vi "Display.vi"() -> ()   [LabVIEW 2020]
panel:
  in  "Stop":bool
  in  "Down":bool
  in  "Right":bool
  in  "Left":bool
  in  "Up":bool
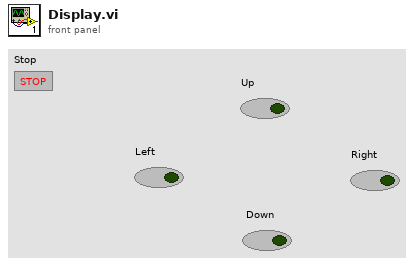
[diagram p1: front panel]
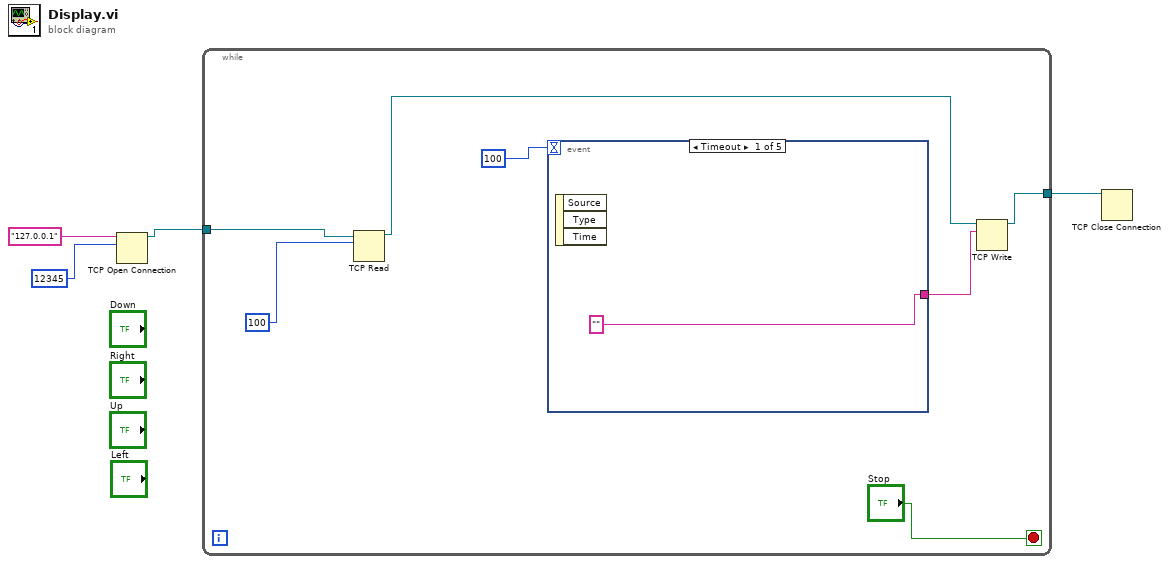
[diagram p0: block diagram]
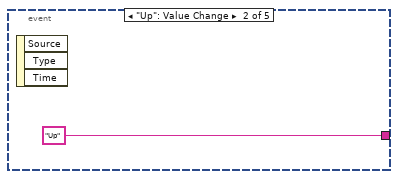
[diagram p2: hidden frame]
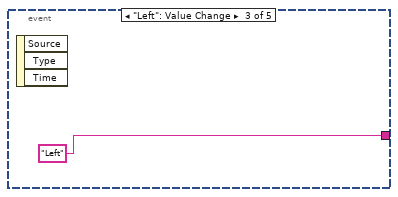
[diagram p3: hidden frame]
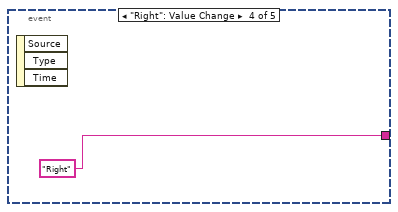
[diagram p4: hidden frame]
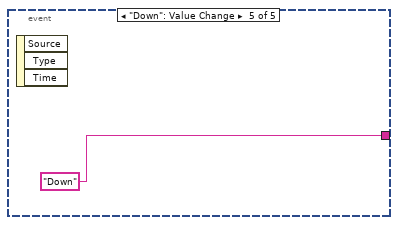
[diagram p5: hidden frame]
diagram:
  n1 = TCP Open Connection(address="127.0.0.1", remote port or service name=12345) -> (connection ID=w2:refnum<k5>)  [unwired: 3 in, 1 out]
  n2 = while {
    tunnel: w2 -> [w10]
    tunnel: [w8] -> w1
    stop <- "Stop" stop-if-true
    n3 = TCP Read(connection ID=w10, bytes to read=100) -> (connection ID out=w9:refnum<k5>)  [unwired: 3 in, 2 out]
    n4 = event shown="[0] Timeout" {
      selector: _ -> [_ _ _ _ _]
      dyn-events: _ -> [_ _ _ _ _]
      timeout: 100 -> [_ _ _ _ _]
      tunnel: ["" "Up" "Left" "Right" "Down"] -> w7
      event Timeout {
        n5 = event-data() -> ()  [unwired: 1 in, 3 out]
      }
      event "Up": Value Change {
        n6 = event-data() -> ()  [unwired: 1 in, 3 out]
      }
      event "Left": Value Change {
        n7 = event-data() -> ()  [unwired: 1 in, 3 out]
      }
      event "Right": Value Change {
        n8 = event-data() -> ()  [unwired: 1 in, 3 out]
      }
      event "Down": Value Change {
        n9 = event-data() -> ()  [unwired: 1 in, 3 out]
      }
    }
    n10 = TCP Write(connection ID=w9, data in=w7) -> (connection ID out=w8:refnum<k5>)  [unwired: 2 in, 2 out]
  }
  n11 = TCP Close Connection(connection ID=w1) -> ()  [unwired: 2 in, 2 out]
